vi "Unreserve Sessions Impl.vi"(8 "error in":errorcluster, 11 "data in":T1) -> (0 "error out":errorcluster, 3 "data out":T1)   [LabVIEW 2020, in "MeasurementLink Session Management.lvlib" / "Session Reservation.lvclass"]
uses:
  Session Reservation.lvclass
  Data.ctl
  Connection Map/Connection Map.lvclass
  IState/IState.lvclass
  Session and Driver Info.ctl
  MeasurementLink Instrument/IInstrument/IInstrument.lvclass
  MeasurementLink Session Management Client/RPC Messages/ni_measurementlink_sessionmanagement_v1_SessionInformation.ctl
  MeasurementLink Session Management Client/RPC Messages/nidevice_grpc_Session.ctl
  MeasurementLink Session Management Client/RPC Messages/ni_measurementlink_sessionmanagement_v1_ChannelMapping.ctl
  MeasurementLink Session Management Client/RPC Messages/ni_measurementlink_PinMapContext.ctl
  MeasurementLink gRPC Utilities/gRPC Client Pool/FGV Action.ctl
  MeasurementLink Session Management Client/RPC Messages/ni_measurementlink_sessionmanagement_v1_UnreserveSessionsRequest.ctl
  Unreserved State/Unreserved State.lvclass
  C:/dev/measurementlink-labview/Source/Runtime/MeasurementLink Session Management/IState/IState.lvclass
  Session Reservation.lvclass/Session Reservation.ctl
  MeasurementLink Session Management Client/MeasurementLink Session Management Client.lvlib
  MeasurementLink gRPC Utilities/gRPC Client Pool/gRPC Client Pool.lvclass
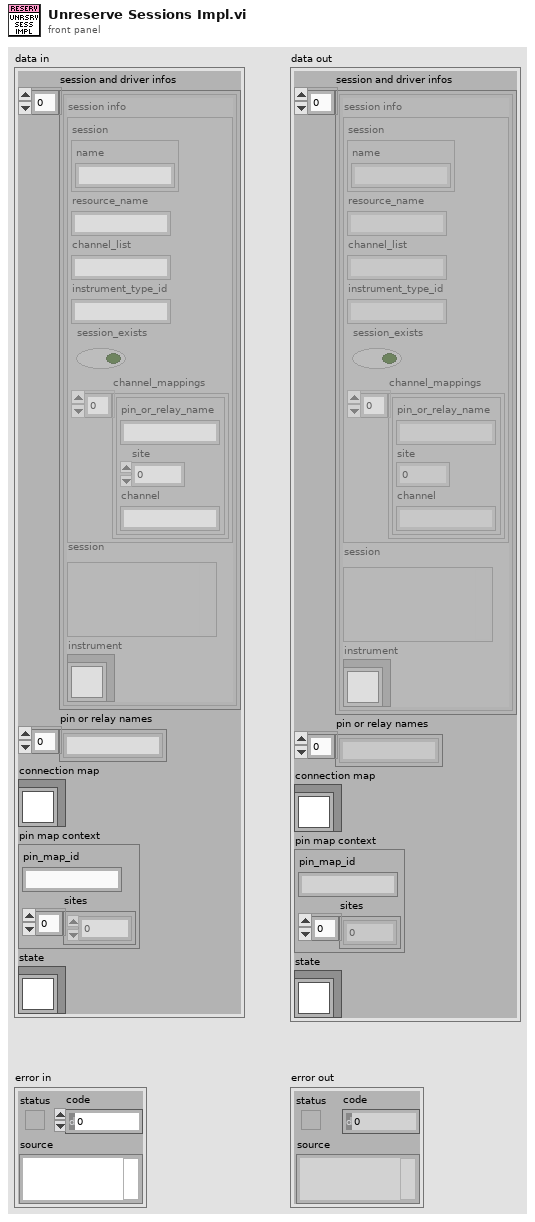
[diagram p1: front panel]
types:
  T1 = typedef "MeasurementLink Session Management.lvlib/Session Reservation.lvclass/Data.ctl" = cluster{"session and driver infos":T2[], "pin or relay names":string[], "connection map":refnum<class "Connection Map.lvclass">, "pin map context":T6, "state":refnum<class "IState.lvclass">}
  T2 = typedef "MeasurementLink Session Management.lvlib/Session Reservation.lvclass/Session and Driver Info.ctl" = cluster{"session info":T3, "session":variant, "instrument":refnum<class "IInstrument.lvclass">}
  T3 = typedef "MeasurementLink Session Management Client.lvlib/ni_measurementlink_sessionmanagement_v1_SessionInformation.ctl" = cluster{"session":T4, "resource_name":string, "channel_list":string, "instrument_type_id":string, "session_exists":bool, "channel_mappings":T5[]}
  T4 = typedef "MeasurementLink Session Management Client.lvlib/nidevice_grpc_Session.ctl" = cluster{"name":string}
  T5 = typedef "MeasurementLink Session Management Client.lvlib/ni_measurementlink_sessionmanagement_v1_ChannelMapping.ctl" = cluster{"pin_or_relay_name":string, "site":i32, "channel":string}
  T6 = typedef "MeasurementLink Session Management Client.lvlib/ni_measurementlink_PinMapContext.ctl" = cluster{"pin_map_id":string, "sites":i32[]}
  T7 = typedef "MeasurementLink Session Management Client.lvlib/ni_measurementlink_sessionmanagement_v1_UnreserveSessionsRequest.ctl" = cluster{"sessions":T3[]}
  T8 = typedef "MeasurementLink gRPC Utilities.lvlib/gRPC Client Pool.lvclass/FGV Action.ctl" = enum16{"Get Discovery Client", "Get Session Client", "Get Pinmap Client", "Destroy Clients"}
  T9 = typedef "grpc-lvsupport-release.lvlib/grpcId.ctl" = u64
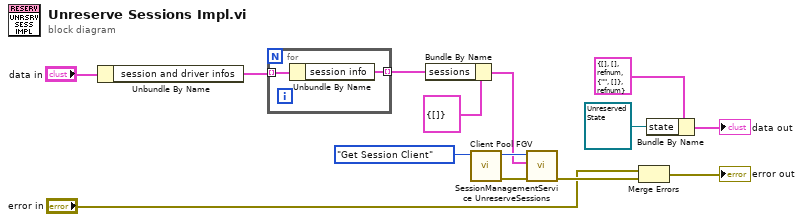
[diagram p0: block diagram]
diagram:
  n1 = Unbundle By Name("data in") -> ("session and driver infos"=w5:T2[])
  n2 = for {
    tunnel: w5 -> [w16] mode=indexing
    tunnel: [w15] -> w7 mode=indexing
    n3 = Unbundle By Name(w16) -> ("session info"=w15:T3)
  }
  n4 = Bundle By Name(cluster=T7 {"sessions"=[]} ("Request Data"), "sessions"=w7) -> (w6:T7)
  n5 = call "Client Pool FGV.vi"("Action"=FGV_Action."Get Session Client") -> ("error out"=w10:errorcluster, "grpc client id"=w9:T9)  [unwired: 9 in]
  n6 = call "SessionManagementService UnreserveSessions.vi"("error in"=w10, "Request Data"=w6, "gRPC ID"=w9) -> ("error out"=w14:errorcluster)  [unwired: 6 in, 2 out]
  n7 = Merge Errors("error in", w14) -> (→"error out":errorcluster)
  n8 = Bundle By Name(cluster=T1 {"session and driver infos"=[], "pin or relay names"=[], "connection map"=refnum, "pin map context"={"pin_map_id"="", "sites"=[]}, "state"=refnum} ("data out"), "state"=refnum<class "Unreserved State.lvclass"> refnum ("MeasurementLink Session Management.lvlib:Unreserved State.lvclass")) -> (→"data out":T1)
